vi "Revert Main.vi"() -> ()   [LabVIEW 2013, in "LVH-Revert.lvlib"]
uses:
  LVH-Revert.lvlib
  Type Defs/Revert Worker State.ctl
  <vilib>/National Instruments/LabVIEW Interface for Amazon S3/Typedefs/AMZ_S3_API_PUT Object Request Parameters.ctl
  <vilib>/National Instruments/LabVIEW Interface for Amazon S3/Typedefs/AMZ_S3_ACL.ctl
  <vilib>/National Instruments/LabVIEW Interface for Amazon S3/Typedefs/AMZ_S3_Storage Class.ctl
  <vilib>/National Instruments/LabVIEW Interface for Amazon S3/Typedefs/AMZ_S3_Object Metadata.ctl
  <vilib>/National Instruments/LabVIEW 2012 AWS Toolkit/SQS/VI Source/Public Typedefs/AWS_SQS SendMessage.ctl
  <vilib>/National Instruments/LabVIEW 2012 AWS Toolkit/SQS/VI Source/AWS SQS Class/AWS_SQS.lvclass
  <vilib>/National Instruments/LabVIEW Interface for Amazon S3/LV Interface for Amazon S3.lvlib
  <vilib>/National Instruments/LabVIEW 2012 AWS Toolkit/SQS/VI Source/AWS_SQS.lvlib
  <vilib>/LabVIEW Hacker/LVH-Toolbox/Common/LVH-Common.lvlib
panel:
  out "Jobs Processed":i32
  out "Error Out":errorcluster
  out "Iteration":i32
  out "Body":string
  in  "Stop Button":bool
  # "MAIN"
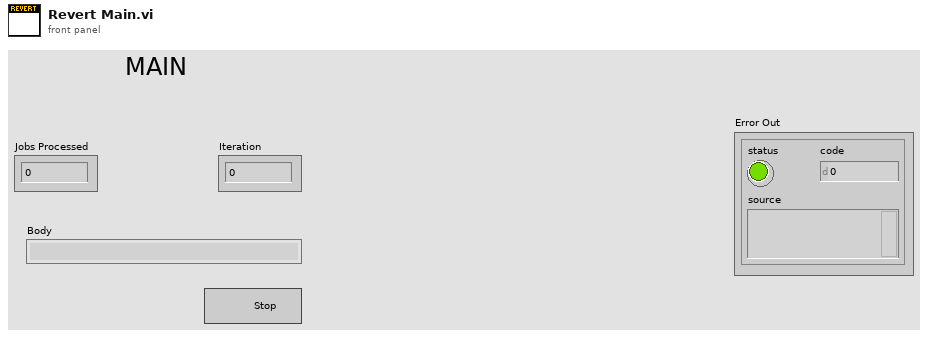
[diagram p1: front panel]
types:
  T1 = typedef "LVH-Revert.lvlib/Revert Worker State.ctl" = enum16{"Poll For Job", "Get Source", "Revert", "Upload Files", "Notify User"}
  T2 = typedef "LVH-Revert.lvlib/Revert Worker Config.ctl" = cluster{"Job Queue":refnum<class "AWS_SQS.lvclass">, "Job Done Queue":refnum<class "AWS_SQS.lvclass">, "Source File Name":string, "Output Path":string, "Source Directory":path, "Unzip Directory":path, "Backsave Directory":path, "Output Directory":path, "LabVIEW Version":T3}
  T3 = typedef "LVH-Toolbox.lvlib/LVH-Common.lvlib/LabVIEW Version.ctl" = enum16{"8.0", "8.2", "8.6", "9.0", "10.0", "11.0", "12.0", "13.0"}
  T4 = enum16{"open", "replace", "create", "open or create", "replace or create", "replace or create with confirmation"}
  T5 = typedef "LV Interface for Amazon S3.lvlib/AMZ_S3_API_PUT Object Request Parameters.ctl" = cluster{"Content Type":string, "ACL":T6, "Storage Class":T7, "User Metadata":T8[], "Content MD5":string}
  T6 = typedef "LV Interface for Amazon S3.lvlib/AMZ_S3_ACL.ctl" = enum16{"private", "public-read", "public-read-write", "authenticated-read", "bucket-owner-read", "bucket-owner-full-control"}
  T7 = typedef "LV Interface for Amazon S3.lvlib/AMZ_S3_Storage Class.ctl" = enum16{"STANDARD", "REDUCED_REDUNDANCY"}
  T8 = typedef "LV Interface for Amazon S3.lvlib/AMZ_S3_Object Metadata.ctl" = cluster{"Key":string, "Value":string}
  T9 = typedef "AWS_SQS.lvlib/AWS_SQS SendMessage.ctl" = cluster{"MessageBody":string, "DelaySeconds":i32}
  T10 = typedef "AWS_SQS.lvlib/ReceiveMesageResult.ctl" = cluster{"Body":string, "MD5OfBody":string, "MessageId":string, "ReceiptHandle":string, "Attributes":cluster{"AttributeName":string, "AttributeValue":string}[]}
  T11 = typedef "LVH-Revert.lvlib/Revert Config.ctl" = cluster{"Revert Paths":T12, "LabVIEW Files":T13, "LabVIEW Version":T3}
  T12 = typedef "LVH-Revert.lvlib/Paths.ctl" = cluster{"Archive Path":path, "Unzip Directory":path, "Backsave Directory":path, "Output Archive":path, "Backsave Common Directory":path}
  T13 = typedef "LVH-Revert.lvlib/LabVIEW Files.ctl" = cluster{"Projects":path[], "Libraries":path[], "Classes":path[], "XControls":path[], "VIs and Controls":path[], "Non LV Files":path[]}
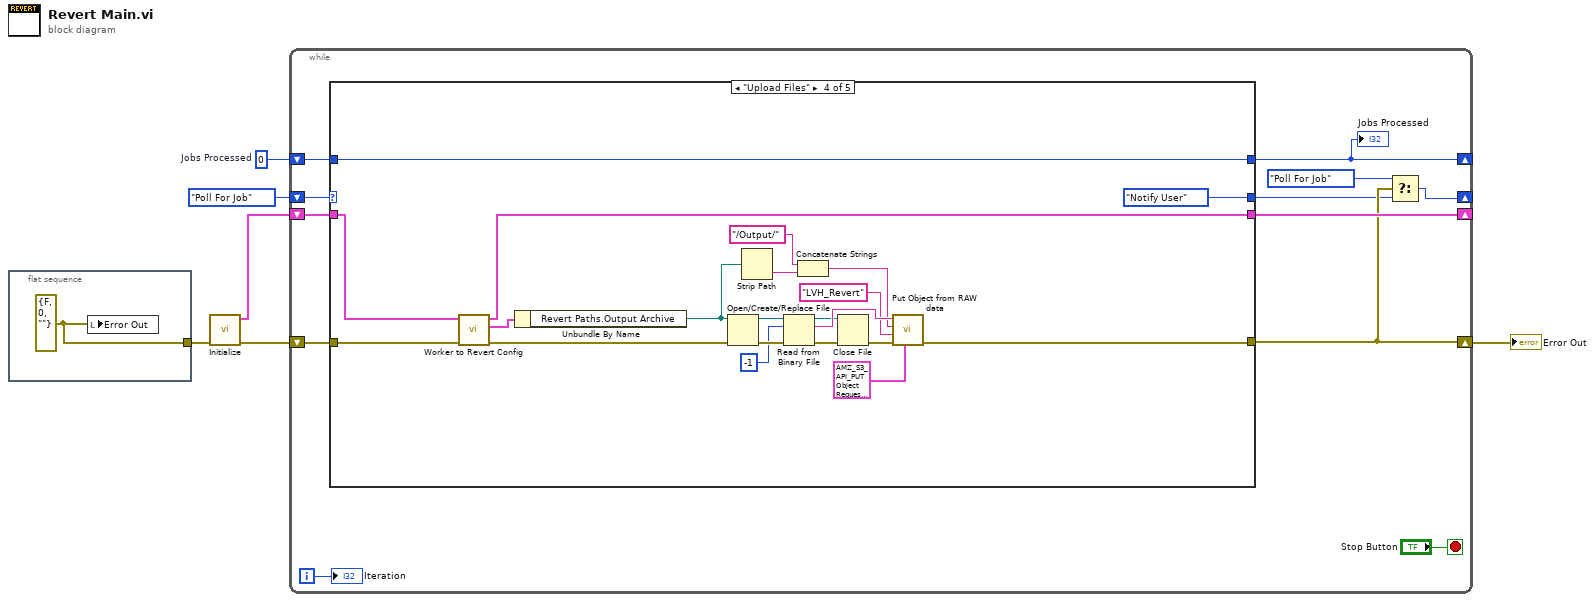
[diagram p0: block diagram]
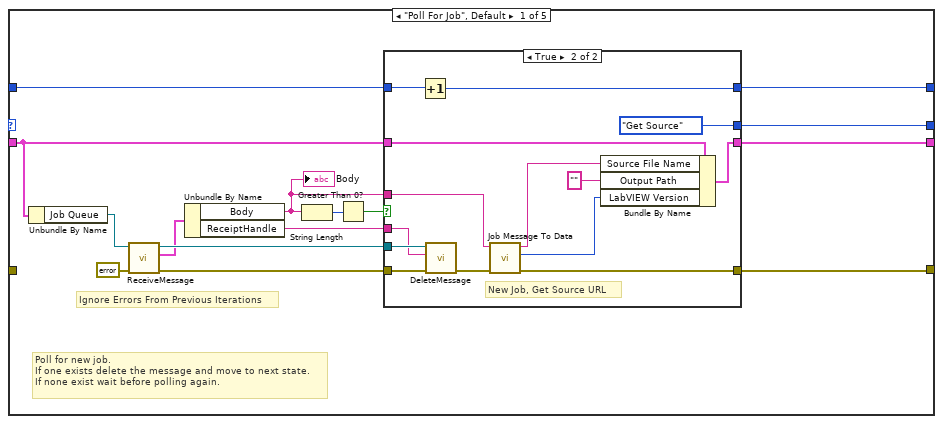
[diagram p2: hidden frame]
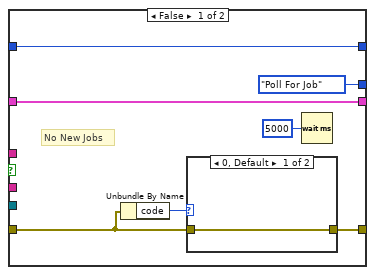
[diagram p3: hidden frame]
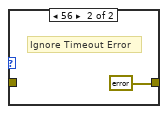
[diagram p4: hidden frame]
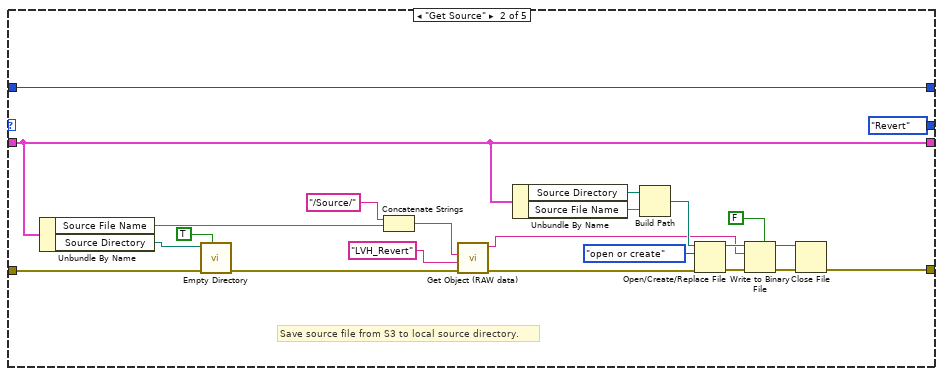
[diagram p5: hidden frame]
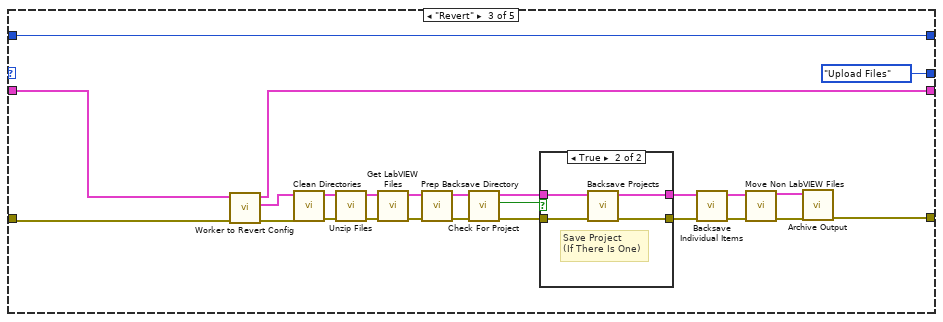
[diagram p6: hidden frame]
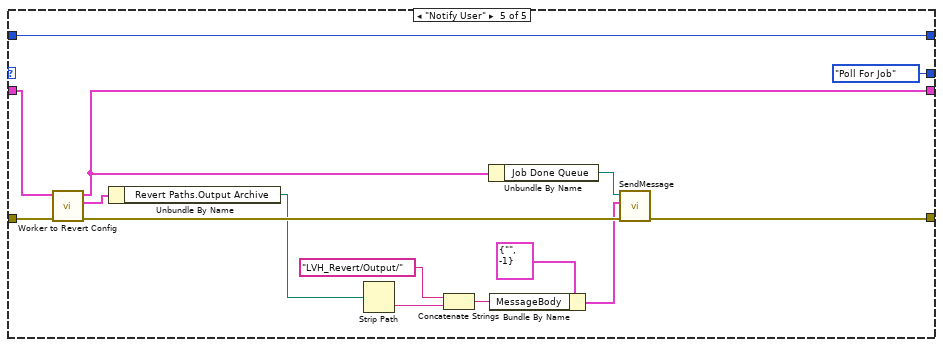
[diagram p8: hidden frame]
diagram:
  w3 = 0  # Jobs Processed
  n1 = flat-sequence {
    tunnel: [w7] -> w1
    frame #0 {
      w7 = errorcluster {"status"=FALSE, "code"=0, "source"=""} ("error constant")
      n2 = local write "Error Out"(w7) -> ()
    }
  }
  n3 = call "Initialize.vi"("Error In"=w1) -> ("Error Out"=w5:errorcluster, "Revert Worker Config"=w4:T2)  [unwired: 9 in]
  n4 = while {
    shift-right: [w9] -> _
    shift-left: Revert_Worker_State."Poll For Job" ("Revert Worker State") -> [w19]
    shift-right: [w12] -> w2
    shift-left: w5 -> [w13]
    shift-right: [w17] -> _
    shift-left: w4 -> [w18]
    shift-right: [w14] -> _
    shift-left: w3 -> [w15]
    i -> [w16]
    stop <- "Stop Button" stop-if-true
    n5 = case shown="\"Upload Files\"" w19 {
      tunnel: w13 -> [_ w66 w87 w119 w146]
      tunnel: [w24 w68 w88 w121 w135] -> w12
      tunnel: w18 -> [w25 w76 w86 w116 w145]
      tunnel: [w27 Revert_Worker_State."Revert" ("Revert Worker State") Revert_Worker_State."Upload Files" ("Revert Worker State") Revert_Worker_State."Notify User" ("Revert Worker State") Revert_Worker_State."Poll For Job" ("Revert Worker State")] -> w10
      tunnel: [w26 w76 w85 w115 w144] -> w17
      tunnel: w15 -> [w22 w59 w81 w112 w133]
      tunnel: [w21 w59 w81 w112 w133] -> w14
      frame "Poll For Job", Default {
        # "Ignore Errors From Previous Iterations"
        # "Poll for new job.\nIf one exists delete the message and move to next state.\nIf none exist wait before polling again."
        n6 = Unbundle By Name(w25) -> ("Job Queue"=w28:refnum<class "AWS_SQS.lvclass">)
        n7 = call <vilib>:"ReceiveMessage.vi"("error in (no error)"=errorcluster {"status"=FALSE, "code"=0, "source"=""}, "AWS_SQS.lvlib:AWS_SQS.lvclass"=w28) -> ("error out"=w32:errorcluster, "Message"=w29:T10, "AWS_SQS.lvlib:AWS_SQS.lvclass"=w33:refnum<class "AWS_SQS.lvclass">)  [unwired: 7 in]
        n8 = Unbundle By Name(w29) -> ("Body"=w23:string, "ReceiptHandle"=w34:string)
        "Body" <- w23
        n9 = String Length(string=w23) -> (length=w30:i32)
        n10 = Greater Than 0?(x=w30) -> (x > 0?=w31:bool)
        n11 = case shown="True" w31 {
          tunnel: w32 -> [w36 w57]
          tunnel: [w37 w47] -> w24
          tunnel: w33 -> [_ w56]
          tunnel: w34 -> [_ w55]
          tunnel: [Revert_Worker_State."Poll For Job" ("Revert Worker State") Revert_Worker_State."Get Source" ("Revert Worker State")] -> w27
          tunnel: [w39 w51] -> w26
          tunnel: w25 -> [w39 w52]
          tunnel: w23 -> [_ w46]
          tunnel: w22 -> [w35 w45]
          tunnel: [w35 w44] -> w21
          frame False {
            # "No New Jobs"
            n12 = Unbundle By Name(w36) -> ("code"=w38:i32)
            n13 = case shown="0, Default" w38 {
              tunnel: [w42 errorcluster {"status"=FALSE, "code"=0, "source"=""} ("error out")] -> w37
              tunnel: w36 -> [w42 _]
              frame 0, Default {
              }
              frame 56 {
                # "Ignore Timeout Error"
              }
            }
            n14 = Wait (ms)(milliseconds to wait=u32 5000) -> ()  [unwired: 1 out]
          }
          frame True {
            # "New Job, Get Source URL"
            n15 = Increment(x=w45) -> (x+1=w44:i32)
            n16 = call <vilib>:"DeleteMessage.vi"("error in (no error)"=w57, "ReceiptHandle"=w55, "AWS_SQS.lvlib:AWS_SQS.lvclass"=w56) -> ("error out"=w50:errorcluster)  [unwired: 5 in, 3 out]
            n17 = call "Job Message To Data.vi"("Error In"=w50, "Job Message"=w46) -> ("Error Out"=w47:errorcluster, "LabVIEW Version"=w48:T3, "Job Source File Name"=w49:string)  [unwired: 7 in]
            n18 = Bundle By Name(cluster=w52, "Source File Name"=w49, "Output Path"="" ("Output URL"), "LabVIEW Version"=w48) -> (w51:T2)
          }
        }
      }
      frame "Get Source" {
        # "Save source file from S3 to local source directory."
        n19 = Unbundle By Name(w76) -> ("Source File Name"=w73:string, "Source Directory"=w64:path)
        n20 = call <vilib>:"Empty Directory.vi"("Delete Files Without Prompt? (F)"=TRUE, "Error In"=w66, "Directory"=w64) -> ("Error Out"=w65:errorcluster)  [unwired: 6 in, 2 out]
        n21 = Concatenate Strings("/Source/" ("string"), w73) -> (w61:string)
        n22 = call <vilib>:"Get Object (RAW data).vi"("error in (no error)"=w65, "Bucket"="LVH_Revert" ("Path"), "Path"=w61) -> ("error out"=w77:errorcluster, "Data"=w69:string)  [unwired: 6 in, 1 out]
        n23 = Unbundle By Name(w76) -> ("Source Directory"=w74:path, "Source File Name"=w72:string)
        n24 = Build Path(base path=w74, name or relative path=w72) -> (appended path=w75:path)
        n25 = Open/Create/Replace File(file path (use dialog)=w75, error in=w77, operation (0:open)=T4."open or create") -> (refnum out=w71:refnum<file>, error out=w79:errorcluster)  [unwired: 3 in, 1 out]
        n26 = Write to Binary File(file (use dialog)=w71, data=w69, error in=w79, 5:FALSE ("prepend array or string size? (T)")) -> (refnum out=w70:refnum<file>, error out=w78:errorcluster)  [unwired: 2 in, 1 out]
        n27 = Close File(refnum=w70, error in=w78) -> (error out=w68:errorcluster)  [unwired: 1 out]
      }
      frame "Revert" {
        n28 = call "Worker to Revert Config.vi"("Error In"=w87, "Revert Worker Config"=w86) -> ("Error Out"=w84:errorcluster, "Revert Config"=w83:T11, "Revert Worker Config"=w85:T2)  [unwired: 7 in]
        n29 = call "Clean Directories.vi"("Error In"=w84, "Revert Config"=w83) -> ("Error Out"=w104:errorcluster, "Revert Config"=w105:T11)  [unwired: 8 in]
        n30 = call "Unzip Files.vi"("Error In"=w104, "Revert Config"=w105) -> ("Error Out"=w102:errorcluster, "Revert Config"=w103:T11)  [unwired: 7 in, 1 out]
        n31 = call "Get LabVIEW Files.vi"("Error In"=w102, "Revert Config"=w103) -> ("Error Out"=w100:errorcluster, "Revert Config"=w101:T11)  [unwired: 8 in]
        n32 = call "Prep Backsave Directory.vi"("Error In"=w100, "Revert Config"=w101) -> ("Error Out"=w99:errorcluster, "Revert Config"=w98:T11)  [unwired: 8 in]
        n33 = call "Check For Project.vi"("Error In"=w99, "Revert Config"=w98) -> ("Error Out"=w96:errorcluster, "Contains Project?"=w95:bool, "Revert Config"=w97:T11)  [unwired: 7 in]
        n34 = case shown="True" w95 {
          tunnel: w97 -> [w106 w111]
          tunnel: w96 -> [w107 w110]
          tunnel: [w107 w109] -> w94
          tunnel: [w106 w108] -> w93
          frame False {
          }
          frame True {
            # "Save Project \n(If There Is One)"
            n35 = call "Backsave Projects.vi"("Error In"=w110, "Revert Config"=w111) -> ("Error Out"=w109:errorcluster, "Revert Config"=w108:T11)  [unwired: 8 in]
          }
        }
        n36 = call "Backsave Individual Items.vi"("Error In"=w94, "Revert Config"=w93) -> ("Error Out"=w92:errorcluster, "Revert Config"=w91:T11)  [unwired: 8 in]
        n37 = call "Move Non LabVIEW Files.vi"("Error In"=w92, "Revert Config"=w91) -> ("Error Out"=w90:errorcluster, "Revert Config"=w89:T11)  [unwired: 8 in]
        n38 = call "Archive Output.vi"("Error In"=w90, "Revert Config"=w89) -> ("Error Out"=w88:errorcluster)  [unwired: 8 in, 1 out]
      }
      frame "Upload Files" {
        n39 = call "Worker to Revert Config.vi"("Error In"=w119, "Revert Worker Config"=w116) -> ("Error Out"=w118:errorcluster, "Revert Config"=w120:T11, "Revert Worker Config"=w115:T2)  [unwired: 7 in]
        n40 = Unbundle By Name(w120) -> ("Revert Paths.Output Archive"=w117:path)
        n41 = Open/Create/Replace File(file path (use dialog)=w117, error in=w118) -> (refnum out=w129:refnum<file>, error out=w130:errorcluster)  [unwired: 4 in, 1 out]
        n42 = Strip Path(path=w117) -> (name=w131:string)  [unwired: 1 out]
        n43 = Read from Binary File(8:w130, 10:-1 ("count (1)"), 11:w129) -> (0:w127:errorcluster, 2:w128:string, 3:w126:refnum<file>)  [unwired: 3 in, 1 out]
        n44 = Concatenate Strings("/Output/" ("string"), w131) -> (w123:string)
        n45 = Close File(refnum=w126, error in=w127) -> (error out=w125:errorcluster)  [unwired: 1 out]
        n46 = call <vilib>:"Put Object from RAW data.vi"("Request Parameters"=T5 {"Content Type"="binary/octet-stream", "ACL"=enum."public-read", "Storage Class"=enum."STANDARD", "User Metadata"=[], "Content MD5"=""}, "error in (no error)"=w125, "Bucket"="LVH_Revert" ("Path"), "Path"=w123, "Data"=w128) -> ("error out"=w121:errorcluster)  [unwired: 5 in, 1 out]
      }
      frame "Notify User" {
        n47 = call "Worker to Revert Config.vi"("Error In"=w146, "Revert Worker Config"=w145) -> ("Error Out"=w142:errorcluster, "Revert Config"=w147:T11, "Revert Worker Config"=w144:T2)  [unwired: 7 in]
        n48 = Unbundle By Name(w147) -> ("Revert Paths.Output Archive"=w138:path)
        n49 = Strip Path(path=w138) -> (name=w139:string)  [unwired: 1 out]
        n50 = Concatenate Strings("LVH_Revert/Output/" ("string"), w139) -> (w137:string)
        n51 = Unbundle By Name(w144) -> ("Job Done Queue"=w143:refnum<class "AWS_SQS.lvclass">)
        n52 = Bundle By Name(cluster=T9 {"MessageBody"="", "DelaySeconds"=-1} ("SendMessage Parameters"), "MessageBody"=w137) -> (w136:T9)
        n53 = call <vilib>:"SendMessage.vi"("error in (no error)"=w142, "SendMessage Parameters"=w136, "AWS_SQS.lvlib:AWS_SQS.lvclass"=w143) -> ("error out"=w135:errorcluster)  [unwired: 6 in, 2 out]
      }
    }
    "Jobs Processed" <- w14
    n54 = Select(t=Revert_Worker_State."Poll For Job", s=w12, f=w10) -> (s? t:f=w9:T1)
    "Iteration" <- w16
  }
  "Error Out" <- w2
